vi "Z900_navX_Internal_ProcessingLoop.vi"(11 "navX Device":T1={"Interface"={"Protocol"=enum."SERIAL", "Update Rate (4Hz-100Hz)"=4, "navX Open TypeDef"=variant}, "Notify Packet"=refnum, "Loop VI Refnum"=refnum, "Ready to Close Occurrence Refnum"=refnum} {"Interface"."Update Rate (4Hz-100Hz)" min=4 max=60 step=1}) -> (0 "error out":errorcluster, 2 "Registry":u8[](array[numeric]))   [LabVIEW 2017, in "navX Library v2.lvlib"]
doc: "This navX VI handles the reading/writing for the navX. All of the good stuff is in here.\nTHIS VI SHOULD NOT BE CALLED BY THE USER!"
uses:
  navX Library v2.lvlib
  TypeDefs/Z900_navX_DeviceTypeDef.ctl
  TypeDefs/Z900_navX_ProtocolTypeDef.ctl
  TypeDefs/Z900_navX_NotifyPacketTypeDef.ctl
  TypeDefs/Z900_navX_ActionTypeDef.ctl
  <vilib>/Platform/TimedLoop/XDataNode/timing_clust.ctl
  <vilib>/Platform/TimedLoop/XDataNode/nitl_modes.ctl
  <vilib>/Platform/TimedLoop/XDataNode/wakeup.ctl
  TypeDefs/navX Open TypeDefs/Z900_navX_OpenTypeDef_Serial.ctl
  NI WPI/WPI_SerialPort_USB.ctl
  TypeDefs/Z900_navX_SerialStreamTypeDef.ctl
  TypeDefs/Z900_navX_ZeroVectorTypeDef.ctl
  TypeDefs/Z900_navX_DeviceRegisters.ctl
  TypeDefs/Flags/Z900_navX_Flags_CapabilityTypeDef.ctl
  <vilib>/Rock Robotics/SystemInterfaces/Utilities/FPGA_UtilitiesRead LocalTime.vi
  <vilib>/Platform/TimedLoop/XDataNode/XDataNode.xnode
  <vilib>/Platform/TimedLoop/XDataNode/XDNodeRunTimeDep.lvlib
  NI WPI/NI WPI Serial USB.lvlib
panel:
  out "Connected":bool
  in  "Halt":bool
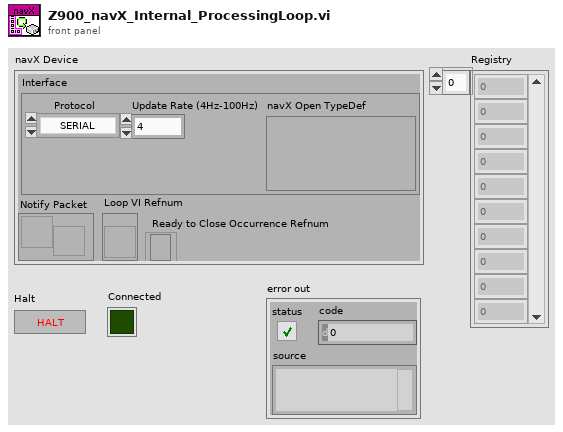
[diagram p1: front panel]
types:
  T1 = typedef "navX Library v2.lvlib/Z900_navX_DeviceTypeDef.ctl" = cluster{"Interface":cluster{"Protocol":T2, "Update Rate (4Hz-100Hz)":u8, "navX Open TypeDef":variant}, "Notify Packet":refnum<notifier>, "Loop VI Refnum":refnum<vi>, "Ready to Close Occurrence Refnum":refnum<k4>}
  T2 = typedef "navX Library v2.lvlib/Z900_navX_ProtocolTypeDef.ctl" = enum16{"SERIAL", "I2C", "SPI"}
  T3 = typedef "navX Library v2.lvlib/Z900_navX_InterfaceTypeDef.ctl" = cluster{"SerialPortRef":T4, "I2CDevRef":T5, "SPIDevRef":T7}
  T4 = typedef "WPI_SerialPortRef.ctl" = cluster{"DevStatus":errorcluster, "Serial Port Name":refnum<visa-resource-name>}
  T5 = typedef "WPI_I2CDevRef.ctl" = cluster{"DevStatus":errorcluster, "Device Address":u8, "Handle":i32, "I2C Bus":T6}
  T6 = typedef "i2c_bus.ctl" = enum16{"I2C On-Board", "I2C MXP", "Invalid"}
  T7 = typedef "WPI_SPIDevRef.ctl" = cluster{"DevStatus":errorcluster, "Handle":i32, "SPI Bus":T8}
  T8 = typedef "spi_bus.ctl" = enum16{"SPI On-Board, CS0", "SPI On-Board, CS1", "SPI On-Board, CS2", "SPI On-Board, CS3", "SPI MXP", "Invalid"}
  T9 = cluster{"Last Valid FPGA Time":dbl, "Error Count":i32, "Initialized":bool}
  T10 = typedef "XDNodeRunTimeDep.lvlib/timing_clust.ctl" = cluster{"Expected End [f-1]":u64, "Actual End [f-1]":u64, "Finished Late? [f-1]":bool, "Expected End [i-1]":u64, "Actual End [i-1]":u64, "Finished Late? [i-1]":bool, "Expected Start [i]":u64, "Actual Start [i]":u64, "Expected Start [f]":u64, "Actual Start [f]":u64, "Source Name":string, "Structure Name":string, "Period":i64, "Deadline":i64, "Offset":i64, "Start":i64, "Priority":i32, "Timeout":i32, "Mode":T11, "Wakeup Reason":T12, "Error":errorcluster, "Source Type":string, "Secondary Source Type":string, "Global End Time":u64, "Global Start Time":u64, "Frame Duration":u64, "Iteration Duration":u64, "Assigned CPU":i32, "I/O Scan Engine Mode":u32}
  T11 = typedef "XDNodeRunTimeDep.lvlib/nitl_modes.ctl" = enum32{"No Change", "Process missed periods, maintain original phase", "Discard missed periods, maintain original phase", "Process missed periods, ignore original phase", "Discard missed periods, ignore original phase"}
  T12 = typedef "XDNodeRunTimeDep.lvlib/wakeup.ctl" = enum32{"Normal", "Aborted", "Asynchronous wakeup", "Timing source error", "Timed loop error", "Timeout"}
  T13 = typedef "navX Library v2.lvlib/Z900_navX_OpenTypeDef_Serial.ctl" = cluster{"Serial Port":T14, "Stream Type":T15}
  T14 = typedef "NI WPI Serial USB.lvlib/WPI_SerialPort_USB.ctl" = enum16{"Onboard RS-232", "MXP TTL", "USB"}
  T15 = typedef "navX Library v2.lvlib/Z900_navX_SerialStreamTypeDef.ctl" = enum16{"YRPH", "Quaterinons", "Gyro/Raw", "AHRS", "AHRSAndPositioning"}
  T16 = typedef "navX Library v2.lvlib/Z900_navX_ZeroVectorTypeDef.ctl" = cluster{"X":bool, "Y":bool, "Z":bool}
  T17 = typedef "navX Library v2.lvlib/Z900_navX_NotifyPacketTypeDef.ctl" = cluster{"navX Action":T18, "Data":variant}
  T18 = typedef "navX Library v2.lvlib/Z900_navX_ActionTypeDef.ctl" = enum16{"None", "Halt", "Update Serial Protocol", "Zero-Yaw", "Zero-Displacement", "Zero-Velocity"}
  T19 = typedef "navX Library v2.lvlib/Z900_navX_DeviceRegisters.ctl" = u8
  T20 = typedef "navX Library v2.lvlib/Z900_navX_Flags_CapabilityTypeDef.ctl" = u16
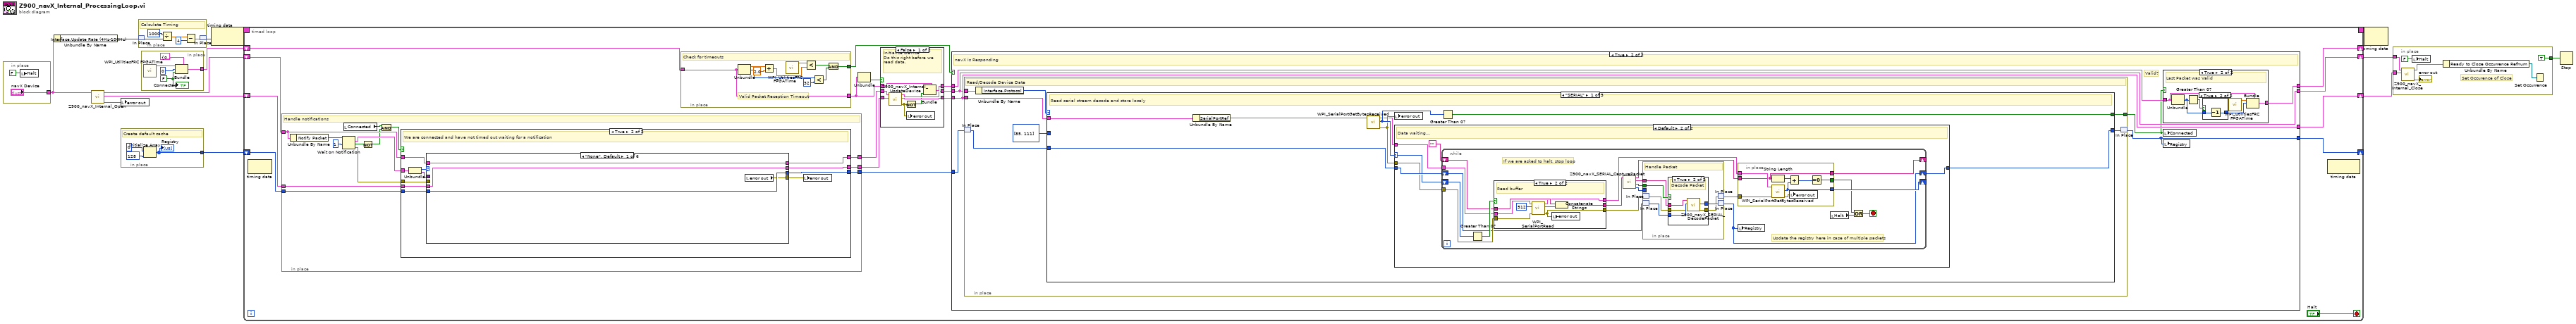
[diagram p0: block diagram]
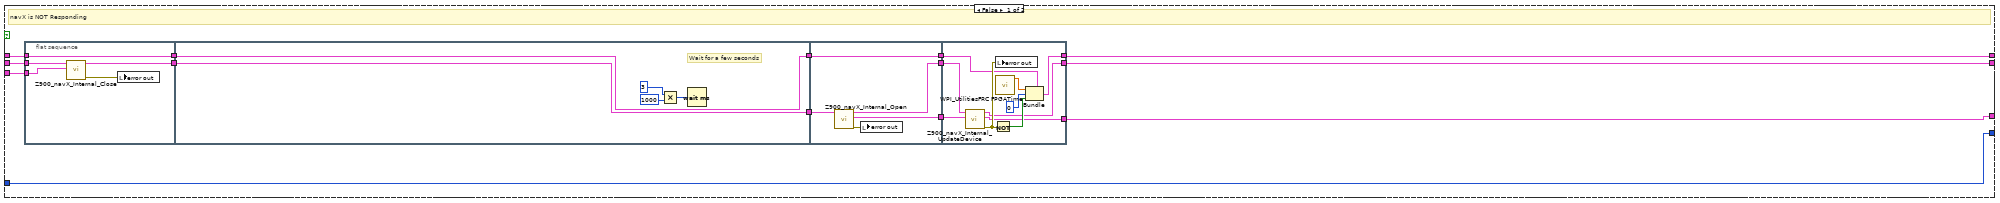
[diagram p3: hidden frame]
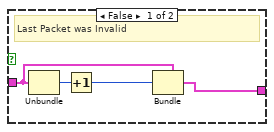
[diagram p4: hidden frame]
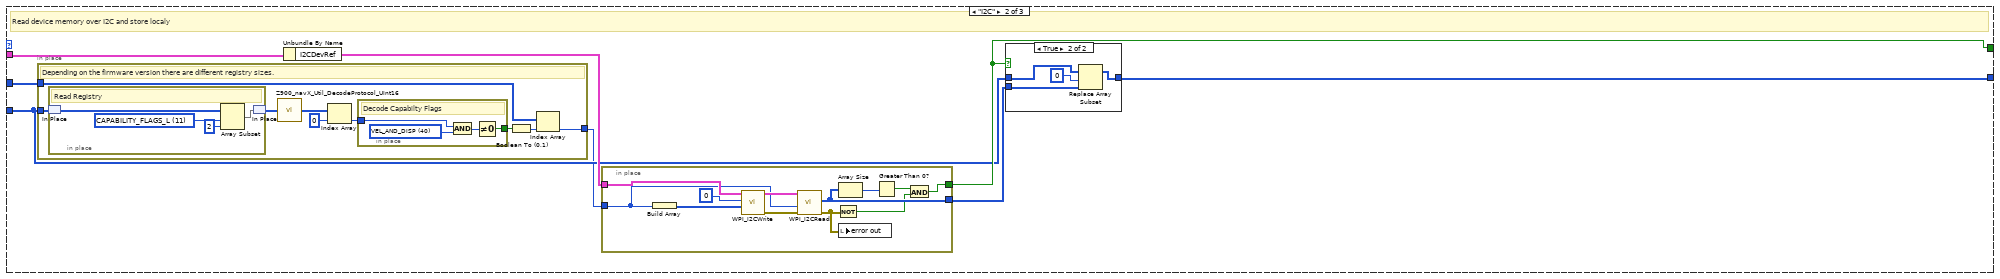
[diagram p9: hidden frame]
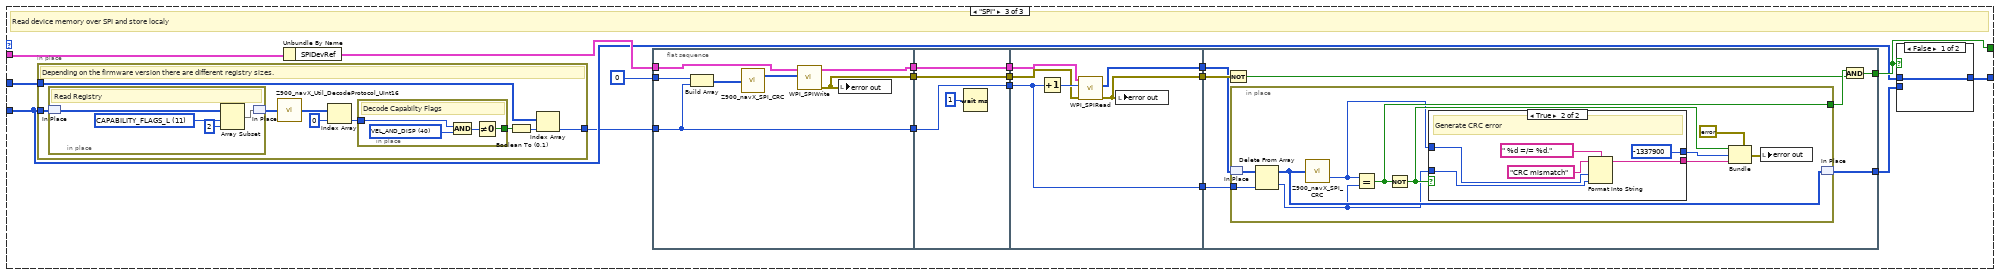
[diagram p11: hidden frame]
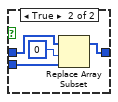
[diagram p12: hidden frame]
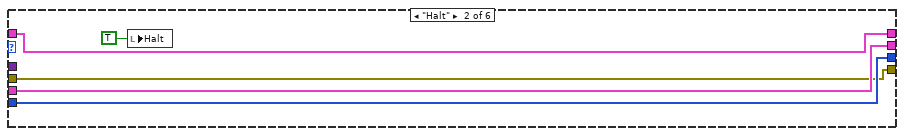
[diagram p15: hidden frame]
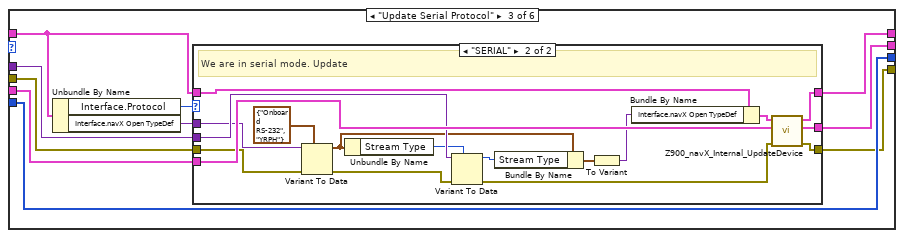
[diagram p16: hidden frame]
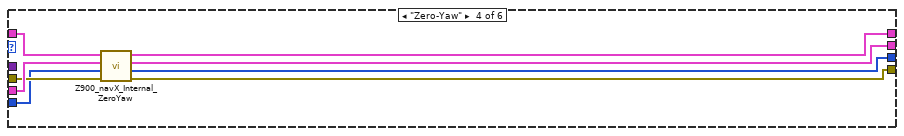
[diagram p18: hidden frame]
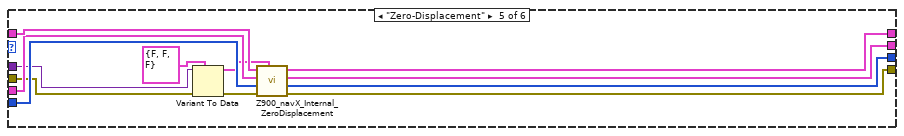
[diagram p19: hidden frame]
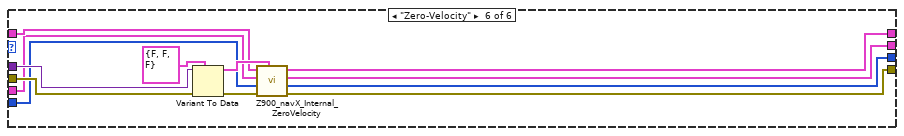
[diagram p20: hidden frame]
diagram:
  n1 = in-place {
    in-place-border: ["navX Device"] -> w6
    n2 = local write "Halt"(FALSE ("Halt")) -> ()
  }
  n3 = Unbundle By Name(w6) -> ("Interface.Update Rate (4Hz-100Hz)"=w10:u8)
  n4 = call "Z900_navX_Internal_Open.vi"("navX Device"=w6) -> ("error out"=w2:errorcluster, "Interface TypeDefs"=w5:T3, "navX Device"=w3:T1)  [unwired: 8 in]
  n5 = local write "error out"(w2) -> ()
  n6 = in-place {
    in-place-border: [w16] -> w9
    # "Create default cache"
    n7 = Initialize Array(u8 0 ("Received Data"), 128 ("hex")) -> (w16:u8[])
    "Registry" <- w16
  }
  n8 = in-place {
    # "Calculate Timing"
    n9 = in-place-match #1(w10) -> (w22:u8)
    n10 = Divide(x=1000, y=w22) -> (x/y=w20:dbl)
    n11 = Subtract(x=w20, y=4) -> (x-y=w19:dbl)
    n12 = in-place-match #1(w19) -> (w11:u8)
  }
  n13 = in-place {
    in-place-border: [w26] -> w4
    w24 = FALSE ("Initialized")
    n14 = call <vilib>:"WPI_UtilitiesFRC FPGATime.vi"() -> ("FPGA Time"=w27:dbl)  [unwired: 10 in, 1 out]
    n15 = Bundle(cluster=T9 {"Last Valid FPGA Time"=0.0, "Error Count"=0, "Initialized"=FALSE}, "Last Valid FPGA Time"=w27, "Error Count"=0, "Initialized"=w24) -> (w26:T9)
    "Connected" <- w24
  }
  n16 = node-c288(w11) -> (w13:T10)
  n17 = timed-loop {
    timing: w13 -> [_]
    timing-out: [_] -> w12
    shift-right: [w46] -> _
    shift-left: w9 -> [w42]
    shift-right: [w43] -> w8
    shift-left: w3 -> [w32]
    shift-right: [w44] -> w7
    shift-left: w5 -> [w31]
    shift-right: [w45] -> _
    shift-left: w4 -> [w29]
    stop <- "Halt" stop-if-true
    n18 = node-c288() -> ()  [unwired: 1 in, 1 out]
    n19 = in-place {
      in-place-border: w32 -> [w334]
      in-place-border: w31 -> [w333]
      in-place-border: [w332] -> w35
      in-place-border: [w331] -> w36
      in-place-border: w42 -> [w329]
      in-place-border: [w328] -> w41
      # "Handle notifications"
      n20 = Unbundle By Name(w334) -> ("Notify Packet"=w336:refnum<notifier>)
      n21 = Wait on Notification(notifier=w336, timeout in ms (-1)=1) -> (notification=w337:T17, timed out?=w327:bool, error out=w330:errorcluster)  [unwired: 2 in, 1 out]
      n22 = local read "Connected"() -> (w325:bool)
      n23 = Not(x=w327) -> (.not. x?=w326:bool)
      n24 = And(x=w325, y=w326) -> (x .and. y?=w324:bool)
      n25 = case shown="True" w324 {
        tunnel: w337 -> [_ w351]
        tunnel: w334 -> [w340 w349]
        tunnel: w333 -> [w339 w348]
        tunnel: [w339 w347] -> w332
        tunnel: [w340 w346] -> w331
        tunnel: w330 -> [_ w344]
        tunnel: w329 -> [w338 w343]
        tunnel: [w338 w342] -> w328
        frame False {
          # "We are either not connected or have timed out waiting for a notification"
        }
        frame True {
          # "We are connected and have not timed out waiting for a notification"
          n26 = Unbundle(w351) -> ("navX Action"=w350:T18, "Data"=w345:variant)
          n27 = case shown="\"None\", Default" w350 {
            tunnel: w349 -> [w355 w360 w364 w398 w410 w417]
            tunnel: w348 -> [w354 w359 w370 w396 w408 w416]
            tunnel: [w354 w359 w369 w395 w406 w413] -> w347
            tunnel: [w355 w360 w368 w397 w407 w414] -> w346
            tunnel: w345 -> [_ _ w367 _ w403 w420]
            tunnel: w344 -> [_ w357 w365 w394 w400 w421]
            tunnel: w343 -> [w353 w358 w363 w393 w409 w415]
            tunnel: [w353 w358 w363 w392 w405 w412] -> w342
            tunnel: [w352 w357 w362 w391 w404 w411] -> w341
            frame "None", Default {
              n28 = local read "error out"() -> (w352:errorcluster)
            }
            frame "Halt" {
              n29 = local write "Halt"(TRUE) -> ()
            }
            frame "Update Serial Protocol" {
              n30 = Unbundle By Name(w364) -> ("Interface.Protocol"=w361:T2, "Interface.navX Open TypeDef"=w366:variant)
              n31 = case shown="\"SERIAL\"" w361 {
                tunnel: w370 -> [w372 w390]
                tunnel: [w372 w389] -> w369
                tunnel: [w373 w388] -> w368
                tunnel: w367 -> [_ w387]
                tunnel: w366 -> [_ w384]
                tunnel: w365 -> [w371 w381]
                tunnel: w364 -> [w373 w380]
                tunnel: [w371 w374] -> w362
                frame Default {
                  # "We don't care if we are not in serial mode."
                }
                frame "SERIAL" {
                  # "We are in serial mode. Update"
                  n32 = Variant To Data(error in=w381, type=T13 {"Serial Port"=enum."Onboard RS-232", "Stream Type"=enum."YRPH"} ("navX Serial Open"), Variant=w384) -> (data=w377:T13, error out=w382:errorcluster)
                  n33 = Unbundle By Name(w377) -> ("Stream Type"=w376:T15)
                  n34 = Variant To Data(error in=w382, type=w376, Variant=w387) -> (data=w375:T15, error out=w386:errorcluster)
                  n35 = Bundle By Name(cluster=w377, "Stream Type"=w375) -> (w385:T13)
                  n36 = To Variant(anything=w385) -> (Variant=w379:variant)
                  n37 = Bundle By Name(cluster=w380, "Interface.navX Open TypeDef"=w379) -> (w378:T1)
                  n38 = call "Z900_navX_Internal_UpdateDevice.vi"("error in (no error)"=w386, "Interface TypeDefs"=w390, "navX Device"=w378) -> ("error out"=w374:errorcluster, "Interface TypeDefs"=w389:T3, "navX Device"=w388:T1)  [unwired: 6 in]
                }
              }
            }
            frame "Zero-Yaw" {
              n39 = call "Z900_navX_Internal_ZeroYaw.vi"("error in (no error)"=w394, "Registry"=w393, "Interface TypeDefs"=w396, "navX Device"=w398) -> ("error out"=w391:errorcluster, "Registry"=w392:u8[], "Interface TypeDefs"=w395:T3, "navX Device"=w397:T1)  [unwired: 4 in]
            }
            frame "Zero-Displacement" {
              n40 = Variant To Data(error in=w400, type=T16 {"X"=FALSE, "Y"=FALSE, "Z"=FALSE} ("Zero Vector"), Variant=w403) -> (data=w401:T16, error out=w399:errorcluster)
              n41 = call "Z900_navX_Internal_ZeroDisplacement.vi"("Zero Vector"=w401, "error in (no error)"=w399, "Registry"=w409, "Interface TypeDefs"=w408, "navX Device"=w410) -> ("error out"=w404:errorcluster, "Registry"=w405:u8[], "Interface TypeDefs"=w406:T3, "navX Device"=w407:T1)  [unwired: 3 in]
            }
            frame "Zero-Velocity" {
              n42 = Variant To Data(error in=w421, type=T16 {"X"=FALSE, "Y"=FALSE, "Z"=FALSE} ("Zero Vector"), Variant=w420) -> (data=w419:T16, error out=w418:errorcluster)
              n43 = call "Z900_navX_Internal_ZeroVelocity.vi"("Zero Vector"=w419, "error in (no error)"=w418, "Registry"=w415, "Interface TypeDefs"=w416, "navX Device"=w417) -> ("error out"=w411:errorcluster, "Registry"=w412:u8[], "Interface TypeDefs"=w413:T3, "navX Device"=w414:T1)  [unwired: 3 in]
            }
          }
          n44 = local write "error out"(w341) -> ()
        }
      }
    }
    n45 = in-place {
      in-place-border: w29 -> [w58]
      in-place-border: [w59] -> w40
      in-place-border: [w58] -> w30
      # "Valid Packet Reception Timeout"
      # "Check for timeouts"
      n46 = Unbundle(w58) -> ("Last Valid FPGA Time"=w67:dbl, "Error Count"=w63:i32)  [unwired: 1 out]
      n47 = Add(x=w67, y=2.0) -> (x+y=w65:dbl)
      n48 = call <vilib>:"WPI_UtilitiesFRC FPGATime.vi"() -> ("FPGA Time"=w64:dbl)  [unwired: 10 in, 1 out]
      n49 = Less?(x=w64, y=w65) -> (x < y?=w61:bool)
      n50 = Less?(x=w63, y=32) -> (x < y?=w60:bool)
      n51 = And(x=w61, y=w60) -> (x .and. y?=w59:bool)
    }
    n52 = Unbundle(w30) -> ("Initialized"=w38:bool)  [unwired: 2 out]
    n53 = case shown="False" w38 {
      tunnel: w30 -> [w54 w57]
      tunnel: [w53 w57] -> w37
      tunnel: w36 -> [w52 w56]
      tunnel: w35 -> [w51 w55]
      tunnel: [w50 w56] -> w33
      tunnel: [w49 w55] -> w34
      frame False {
        # "Initialize Device\nDo this right before we\nread data."
        n54 = call "Z900_navX_Internal_UpdateDevice.vi"("Interface TypeDefs"=w51, "navX Device"=w52) -> ("error out"=w48:errorcluster, "Interface TypeDefs"=w49:T3, "navX Device"=w50:T1)  [unwired: 7 in]
        n55 = Not(x=w48) -> (.not. x?=w47:bool)
        n56 = local write "error out"(w48) -> ()
        n57 = Bundle(cluster=w54, "Initialized"=w47) -> (w53:T9)  [unwired: 2 in]
      }
      frame True {
      }
    }
    n58 = case shown="True" w40 {
      tunnel: w41 -> [w79 w113]
      tunnel: w34 -> [w80 w112]
      tunnel: [w79 w109] -> w46
      tunnel: w37 -> [w68 w111]
      tunnel: [w72 w110] -> w45
      tunnel: w33 -> [w81 w108]
      tunnel: [w73 w108] -> w43
      tunnel: [w76 w112] -> w44
      frame False {
        # "navX is NOT Responding"
        n59 = flat-sequence {
          tunnel: w81 -> [w84]
          tunnel: w80 -> [w86]
          tunnel: [w85] -> w78
          tunnel: [w82] -> w69
          tunnel: w68 -> [w82]
          tunnel: w78 -> [w91]
          tunnel: [w91] -> w77
          tunnel: [w87] -> w70
          tunnel: w69 -> [w87]
          tunnel: w77 -> [w95]
          tunnel: [w96] -> w75
          tunnel: [w94] -> w74
          tunnel: [w92] -> w71
          tunnel: w70 -> [w92]
          tunnel: [w104] -> w72
          tunnel: [w100] -> w76
          tunnel: [w101] -> w73
          tunnel: w71 -> [w99]
          tunnel: w74 -> [w102]
          tunnel: w75 -> [w103]
          frame #0 {
            n60 = call "Z900_navX_Internal_Close.vi"("Interface TypeDefs"=w86, "navX Device"=w84) -> ("error out"=w83:errorcluster, "navX Device"=w85:T1)  [unwired: 8 in]
            n61 = local write "error out"(w83) -> ()
          }
          frame #1 {
            # "Wait for a few seconds"
            n62 = Multiply(x=u32 3 ("milliseconds to wait"), y=u32 1000) -> (x*y=w89:u32)
            n63 = Wait (ms)(milliseconds to wait=w89) -> ()  [unwired: 1 out]
          }
          frame #2 {
            n64 = call "Z900_navX_Internal_Open.vi"("navX Device"=w95) -> ("error out"=w93:errorcluster, "Interface TypeDefs"=w94:T3, "navX Device"=w96:T1)  [unwired: 8 in]
            n65 = local write "error out"(w93) -> ()
          }
          frame #3 {
            n66 = call "Z900_navX_Internal_UpdateDevice.vi"("Interface TypeDefs"=w102, "navX Device"=w103) -> ("error out"=w105:errorcluster, "Interface TypeDefs"=w100:T3, "navX Device"=w101:T1)  [unwired: 7 in]
            n67 = Not(x=w105) -> (.not. x?=w106:bool)
            n68 = local write "error out"(w105) -> ()
            n69 = call <vilib>:"WPI_UtilitiesFRC FPGATime.vi"() -> ("FPGA Time"=w98:dbl)  [unwired: 10 in, 1 out]
            n70 = Bundle(cluster=w99, "Last Valid FPGA Time"=w98, "Error Count"=0, "Initialized"=w106) -> (w104:T9)
          }
        }
      }
      frame True {
        # "Valid?"
        # "navX is Responding"
        n71 = in-place {
          in-place-border: w108 -> [w128]
          in-place-border: w112 -> [w132]
          in-place-border: [w130] -> w107
          # "Read/Decode Device Date"
          n72 = in-place-match #2(w113) -> (w131:u8[])
          n73 = Unbundle By Name(w128) -> ("Interface.Protocol"=w133:T2)
          n74 = case shown="\"SERIAL\"" w133 {
            tunnel: [w139 w206 w253] -> w129
            tunnel: w131 -> [w140 w203 w245]
            tunnel: w132 -> [w141 w208 w260]
            tunnel: [w137 w205 w250] -> w130
            tunnel: i32[] [85, 111] -> [_ w202 w244]
            frame "SERIAL" {
              # "Read serial stream decode and store localy"
              n75 = Unbundle By Name(w141) -> ("SerialPortRef"=w138:T4)
              n76 = call <vilib>:"WPI_SerialPortGetBytesReceived.vi"("SerialPortRef"=w138) -> ("error out"=w135:errorcluster, "Bytes at Port"=w136:u32, "SerialPortRef"=w134:T4)  [unwired: 8 in]
              n77 = local write "error out"(w135) -> ()
              n78 = case shown="Default" w136 {
                selector: w136 -> [_ w143]
                tunnel: [w142 w148] -> w139
                tunnel: w140 -> [w142 w147]
                tunnel: w134 -> [_ w145]
                tunnel: w135 -> [_ w144]
                frame 0 {
                }
                frame Default {
                  # "Data waiting..."
                  n79 = while {
                    shift-right: [w150] -> w148
                    shift-left: w147 -> [w157]
                    shift-right: [w161] -> _
                    shift-left: w143 -> [w168]
                    shift-right: [w160] -> _
                    shift-left: "" -> [w166]
                    tunnel: w145 -> [w165]
                    tunnel: w144 -> [w164]
                    stop <- w153 stop-if-true
                    # "Update the registry here in case of multiple packets"
                    # "If we are asked to halt, stop loop"
                    n80 = Greater Than 0?(x=w168) -> (x > 0?=w167:bool)
                    n81 = case shown="True" w167 {
                      tunnel: w166 -> [w192 w200]
                      tunnel: w165 -> [w191 w199]
                      tunnel: w164 -> [w190 w196]
                      tunnel: [w192 w195] -> w163
                      tunnel: [w191 w194] -> w149
                      tunnel: [w190 w193] -> w156
                      frame False {
                        # "Pass existing buffer"
                      }
                      frame True {
                        # "Read buffer"
                        n82 = call <vilib>:"WPI_SerialPortRead.vi"("error in (no error)"=w196, "Num Bytes to Read"=u32 512, "SerialPortRef"=w199) -> ("error out"=w193:errorcluster, "Buffer"=w198:string, "SerialPortRef"=w194:T4)  [unwired: 6 in]
                        n83 = local write "error out"(w193) -> ()
                        n84 = Concatenate Strings(w200, w198) -> (w195:string)
                      }
                    }
                    n85 = call "Z900_navX_SERIAL_CapturePacket.vi"("Buffer"=w163) -> ("Packet Size"=w158:i32, "Packet Located"=w151:bool, "Packet"=w159:string, "Buffer"=w162:string)  [unwired: 7 in]
                    n86 = in-place {
                      in-place-border: w159 -> [w173]
                      in-place-border: w151 -> [w174]
                      in-place-border: w158 -> [_]
                      # "Handle Packet"
                      n87 = in-place-match #3(w156) -> (w170:errorcluster)
                      n88 = in-place-match #4(w157) -> (w171:u8[])
                      n89 = case shown="True" w174 {
                        tunnel: w173 -> [_ w181]
                        tunnel: [w176 w179] -> w172
                        tunnel: w171 -> [w176 w180]
                        tunnel: w170 -> [w175 w178]
                        tunnel: [w175 w177] -> w169
                        frame False {
                          # "No Packet"
                        }
                        frame True {
                          # "Decode Packet"
                          n90 = call "Z900_navX_SERIAL_DecodePacket.vi"("error in (no error)"=w178, "Data"=w180, "Packet"=w181) -> ("error out"=w177:errorcluster, "Data"=w179:u8[])  [unwired: 6 in, 1 out]
                        }
                      }
                      n91 = in-place-match #3(w169) -> (w155:errorcluster)
                      n92 = in-place-match #4(w172) -> (w150:u8[])
                    }
                    n93 = in-place {
                      in-place-border: w149 -> [w189]
                      in-place-border: w155 -> [w188]
                      in-place-border: w162 -> [w183]
                      in-place-border: [w185] -> w154
                      in-place-border: [w184] -> w161
                      in-place-border: [w183] -> w160
                      n94 = String Length(string=w183) -> (length=w186:i32)
                      n95 = call <vilib>:"WPI_SerialPortGetBytesReceived.vi"("error in (no error)"=w188, "SerialPortRef"=w189) -> ("error out"=w182:errorcluster, "Bytes at Port"=w184:u32)  [unwired: 7 in, 1 out]
                      n96 = Add(x=w186, y=w184) -> (x+y=w187:u32)
                      n97 = local write "error out"(w182) -> ()
                      n98 = Equal To 0?(x=w187) -> (x = 0?=w185:bool)
                    }
                    n99 = local write "Registry"(w150) -> ()
                    n100 = local read "Halt"() -> (w152:bool)
                    n101 = Or(x=w154, y=w152) -> (x .or. y?=w153:bool)
                  }
                }
              }
              n102 = Greater Than 0?(x=w136) -> (x > 0?=w137:bool)
            }
            frame "I2C" {
              # "Read device memory over I2C and store localy"
              n103 = in-place {
                in-place-border: w203 -> [w217]
                in-place-border: w202 -> [w210]
                in-place-border: [w209] -> w201
                # "Depending on the firmware version there are different registry sizes."
                n104 = in-place {
                  w225 = T19 11 items=["WHOAMI"=0, "HW_REV"=1, "FW_VER_MAJOR"=2, "FW_VER_MINOR"=3, "UPDATE_RATE_HZ"=4, "ACCEL_FSR_G"=5, "GYRO_FSR_DPS"=6, "OP_STATUS"=8, "CAL_STATUS"=9, "SELFTEST_STATUS"=10, "CAPABILITY_FLAGS_L"=11, "CAPABILITY_FLAGS_H"=12, "SENSOR_STATUS"=16, "TIMESTAMP"=18, "YAW"=22, "ROLL"=24, "PITCH"=26, "HEADING"=28, "FUSED_HEADING"=30, "ALTITUDE_I"=32, "ALTITUDE_D"=34, "LINERA_ACC_X"=36, "LINERA_ACC_Y"=38, "LINERA_ACC_Z"=40, "QUAT_W"=42, "QUAT_X"=44, "QUAT_Y"=46, "QUAT_Z"=48, "MPU_TEMP_C"=50, "GYRO_X"=52, "GYRO_Y"=54, "GYRO_Z"=56, "ACC_X"=58, "ACC_Y"=60, "ACC_Z"=62, "MAG_X"=64, "MAG_Y"=66, "MAG_Z"=68, "PRESSURE_I"=70, "PRESSURE_D"=72, "PRESSURE_TEMP"=74, "YAW_OFFSET"=76, "QUAT_OFFSET_W"=78, "QUAT_OFFSET_X"=80, "QUAT_OFFSET_Y"=82, "QUAT_OFFSET_Z"=84, "INTEGRATION_CONTROL"=86, "VELOCITY_X"=88, "VELOCITY_Y"=92, "VELOCITY_Z"=96, "DISPLACMENT_X"=100, "DISPLACMENT_Y"=104, "DISPLACEMENT_Z"=108] ("Device Register")
                  # "Read Registry"
                  n105 = in-place-match #5(w217) -> (w223:u8[])
                  n106 = Array Subset(array=w223, index=w225, length=2) -> (w224:u8[])
                  n107 = in-place-match #5(w224) -> (w214:u8[])
                }
                n108 = call "Z900_navX_Util_DecodeProtocol_UInt16.vi"("Little Endian"=w214) -> ("UInt16"=w215:u16[])
                n109 = Index Array(array=w215, index=0) -> (element=w213:u16)
                n110 = in-place {
                  in-place-border: w213 -> [w219]
                  in-place-border: [w218] -> w212
                  w221 = T20 40 items=["OMNIMOUNT"=4, "OMNIMOUNT_CONFIG_MASK"=38, "VEL_AND_DISP"=40, "YAW_RESET"=80] ("Capability Flag")
                  # "Decode Capabilty Flags"
                  n111 = And(x=w219, y=w221) -> (x .and. y?=w220:T20)
                  n112 = Not Equal To 0?(x=w220) -> (x != 0?=w218:bool)
                }
                n113 = Boolean To (0,1)(Boolean=w212) -> (0, 1=w211:i16)
                n114 = Index Array(array=w210, index=w211) -> (element=w209:i32)
              }
              n115 = Unbundle By Name(w208) -> ("I2CDevRef"=w204:T5)
              n116 = in-place {
                in-place-border: [w231] -> w207
                in-place-border: [w230] -> w205
                in-place-border: w204 -> [w228]
                in-place-border: w201 -> [w226]
                n117 = Build Array(w226) -> (w237:i32[])
                n118 = call <vilib>:"WPI_I2CWrite.vi"("I2CDataToSend"=w237, "I2CRegister"=u8 0 ("hex"), "I2CDevRef"=w228) -> ("error out"=w236:errorcluster, "I2CDevRef"=w235:T5)  [unwired: 7 in]
                n119 = call <vilib>:"WPI_I2CRead.vi"("error in (no error)"=w236, "I2CBytesToRead"=w226, "I2CDevRef"=w235) -> ("error out"=w227:errorcluster, "Data Out"=w231:u8[])  [unwired: 6 in, 1 out]
                n120 = Not(x=w227) -> (.not. x?=w229:bool)
                n121 = Array Size(array=w231) -> (size(s)=w233:i32)
                n122 = local write "error out"(w227) -> ()
                n123 = Greater Than 0?(x=w233) -> (x > 0?=w232:bool)
                n124 = And(x=w232, y=w229) -> (x .and. y?=w230:bool)
              }
              n125 = case shown="True" w205 {
                tunnel: w203 -> [w238 w242]
                tunnel: [w238 w241] -> w206
                tunnel: w207 -> [_ w240]
                frame False {
                }
                frame True {
                  n126 = Replace Array Subset(array=w242, new element=w240, index=u8 0 ("hex")) -> (w241:u8[])
                }
              }
            }
            frame "SPI" {
              # "Read device memory over SPI and store localy"
              n127 = in-place {
                in-place-border: w245 -> [w269]
                in-place-border: w244 -> [w262]
                in-place-border: [w261] -> w243
                # "Depending on the firmware version there are different registry sizes."
                n128 = in-place {
                  w277 = T19 11 items=["WHOAMI"=0, "HW_REV"=1, "FW_VER_MAJOR"=2, "FW_VER_MINOR"=3, "UPDATE_RATE_HZ"=4, "ACCEL_FSR_G"=5, "GYRO_FSR_DPS"=6, "OP_STATUS"=8, "CAL_STATUS"=9, "SELFTEST_STATUS"=10, "CAPABILITY_FLAGS_L"=11, "CAPABILITY_FLAGS_H"=12, "SENSOR_STATUS"=16, "TIMESTAMP"=18, "YAW"=22, "ROLL"=24, "PITCH"=26, "HEADING"=28, "FUSED_HEADING"=30, "ALTITUDE_I"=32, "ALTITUDE_D"=34, "LINERA_ACC_X"=36, "LINERA_ACC_Y"=38, "LINERA_ACC_Z"=40, "QUAT_W"=42, "QUAT_X"=44, "QUAT_Y"=46, "QUAT_Z"=48, "MPU_TEMP_C"=50, "GYRO_X"=52, "GYRO_Y"=54, "GYRO_Z"=56, "ACC_X"=58, "ACC_Y"=60, "ACC_Z"=62, "MAG_X"=64, "MAG_Y"=66, "MAG_Z"=68, "PRESSURE_I"=70, "PRESSURE_D"=72, "PRESSURE_TEMP"=74, "YAW_OFFSET"=76, "QUAT_OFFSET_W"=78, "QUAT_OFFSET_X"=80, "QUAT_OFFSET_Y"=82, "QUAT_OFFSET_Z"=84, "INTEGRATION_CONTROL"=86, "VELOCITY_X"=88, "VELOCITY_Y"=92, "VELOCITY_Z"=96, "DISPLACMENT_X"=100, "DISPLACMENT_Y"=104, "DISPLACEMENT_Z"=108] ("Device Register")
                  # "Read Registry"
                  n129 = in-place-match #6(w269) -> (w275:u8[])
                  n130 = Array Subset(array=w275, index=w277, length=2) -> (w276:u8[])
                  n131 = in-place-match #6(w276) -> (w266:u8[])
                }
                n132 = call "Z900_navX_Util_DecodeProtocol_UInt16.vi"("Little Endian"=w266) -> ("UInt16"=w267:u16[])
                n133 = Index Array(array=w267, index=0) -> (element=w265:u16)
                n134 = in-place {
                  in-place-border: w265 -> [w271]
                  in-place-border: [w270] -> w264
                  w273 = T20 40 items=["OMNIMOUNT"=4, "OMNIMOUNT_CONFIG_MASK"=38, "VEL_AND_DISP"=40, "YAW_RESET"=80] ("Capability Flag")
                  # "Decode Capabilty Flags"
                  n135 = And(x=w271, y=w273) -> (x .and. y?=w272:T20)
                  n136 = Not Equal To 0?(x=w272) -> (x != 0?=w270:bool)
                }
                n137 = Boolean To (0,1)(Boolean=w264) -> (0, 1=w263:i16)
                n138 = Index Array(array=w262, index=w263) -> (element=w261:i32)
              }
              n139 = Unbundle By Name(w260) -> ("SPIDevRef"=w246:T7)
              n140 = flat-sequence {
                tunnel: u8 0 ("hex") -> [w289]
                tunnel: w243 -> [w284]
                tunnel: w246 -> [w286]
                tunnel: [w285] -> w259
                tunnel: [w284] -> w256
                tunnel: [w283] -> w249
                tunnel: w259 -> [w292]
                tunnel: [w292] -> w258
                tunnel: [w291] -> w257
                tunnel: w256 -> [w291]
                tunnel: w249 -> [w290]
                tunnel: [w290] -> w248
                tunnel: w258 -> [w299]
                tunnel: w257 -> [w296]
                tunnel: [w297] -> w255
                tunnel: [w296] -> w254
                tunnel: w248 -> [w295]
                tunnel: [w294] -> w247
                tunnel: w255 -> [w302]
                tunnel: w254 -> [w306]
                tunnel: [w303] -> w250
                tunnel: [w301] -> w252
                tunnel: w247 -> [w305]
                frame #0 {
                  n141 = Build Array(w289, w284) -> (w288:i32[])
                  n142 = call "Z900_navX_SPI_CRC.vi"("Message"=w288) -> ("Message with CRC"=w287:u8[])  [unwired: 1 out]
                  n143 = call <vilib>:"WPI_SPIWrite.vi"("Data To Send"=w287, "SPIDevRef"=w286) -> ("error out"=w283:errorcluster, "SPIDevRef"=w285:T7)  [unwired: 7 in, 1 out]
                  n144 = local write "error out"(w283) -> ()
                }
                frame #1 {
                  n145 = Wait (ms)(milliseconds to wait=u32 1) -> ()  [unwired: 1 out]
                }
                frame #2 {
                  n146 = Increment(x=w296) -> (x+1=w298:i32)
                  n147 = call <vilib>:"WPI_SPIRead.vi"("error in (no error)"=w295, "Num to Read"=w298, "SPIDevRef"=w299) -> ("error out"=w294:errorcluster, "Received Data"=w297:u8[])  [unwired: 6 in, 1 out]
                  n148 = local write "error out"(w294) -> ()
                }
                frame #3 {
                  n149 = Not(x=w305) -> (.not. x?=w300:bool)
                  n150 = in-place {
                    in-place-border: w306 -> [w317]
                    in-place-border: [w314] -> w304
                    n151 = in-place-match #7(w302) -> (w316:u8[])
                    n152 = Delete From Array(array=w316, index=w317) -> (deleted portion=w311:u8, array with subset deleted=w315:u8[])  [unwired: 1 in]
                    n153 = call "Z900_navX_SPI_CRC.vi"("Message"=w315) -> ("CRC"=w312:u8)  [unwired: 1 out]
                    n154 = Equal?(x=w312, y=w311) -> (x = y?=w314:bool)
                    n155 = Not(x=w314) -> (.not. x?=w313:bool)
                    n156 = case shown="True" w313 {
                      tunnel: w312 -> [_ w321]
                      tunnel: w311 -> [_ w320]
                      tunnel: [_ w319] -> w310
                      tunnel: [_ -1337900 ("code")] -> w307
                      frame False {
                      }
                      frame True {
                        # "Generate CRC error"
                        n157 = Format Into String(format string=" %d =/= %d.", initial string="CRC mismatch", w321, w320) -> (resulting string=w319:string)  [unwired: 1 in, 1 out]
                      }
                    }
                    n158 = Bundle(cluster=errorcluster {"status"=FALSE, "code"=0, "source"=""} ("error constant"), "status"=w313, "code"=w307, "source"=w310) -> (w308:errorcluster)
                    n159 = local write "error out"(w308) -> ()
                    n160 = in-place-match #7(w315) -> (w301:u8[])
                  }
                  n161 = And(x=w304, y=w300) -> (x .and. y?=w303:bool)
                }
              }
              n162 = case shown="False" w250 {
                tunnel: w245 -> [w278 w282]
                tunnel: [w278 w281] -> w253
                tunnel: w252 -> [_ w280]
                frame False {
                }
                frame True {
                  n163 = Replace Array Subset(array=w282, new element=w280, index=u8 0 ("hex")) -> (w281:u8[])
                }
              }
            }
          }
          n164 = in-place-match #2(w129) -> (w109:u8[])
        }
        n165 = case shown="True" w107 {
          tunnel: [w114 w122] -> w110
          tunnel: w111 -> [w115 w121]
          frame False {
            # "Last Packet was Invalid"
            n166 = Unbundle(w115) -> ("Error Count"=w116:i32)  [unwired: 2 out]
            n167 = Increment(x=w116) -> (x+1=w117:i32)
            n168 = Bundle(cluster=w115, "Error Count"=w117) -> (w114:T9)  [unwired: 2 in]
          }
          frame True {
            # "Last Packet was Valid"
            n169 = Unbundle(w121) -> ("Error Count"=w119:i32)  [unwired: 2 out]
            n170 = Greater Than 0?(x=w119) -> (x > 0?=w120:bool)
            n171 = case shown="True" w120 {
              tunnel: [w124 w125] -> w118
              tunnel: w119 -> [w124 w126]
              frame False {
              }
              frame True {
                n172 = Decrement(x=w126) -> (x-1=w125:i32)
              }
            }
            n173 = call <vilib>:"WPI_UtilitiesFRC FPGATime.vi"() -> ("FPGA Time"=w123:dbl)  [unwired: 10 in, 1 out]
            n174 = Bundle(cluster=w121, "Last Valid FPGA Time"=w123, "Error Count"=w118) -> (w122:T9)  [unwired: 1 in]
          }
        }
        n175 = local write "Connected"(w107) -> ()
        n176 = local write "Registry"(w109) -> ()
      }
    }
    n177 = node-c288() -> ()  [unwired: 1 in, 1 out]
  }
  n178 = node-c288(w12) -> ()  [unwired: 1 out]
  n179 = in-place {
    in-place-border: w8 -> [w431]
    in-place-border: w7 -> [w430]
    in-place-border: [TRUE] -> w1
    # "Set Occurence of Close"
    n180 = call "Z900_navX_Internal_Close.vi"("Interface TypeDefs"=w430, "navX Device"=w431) -> ("error out"=→"error out":errorcluster, "navX Device"=w425:T1)  [unwired: 8 in]
    n181 = local write "Halt"(FALSE ("Halt")) -> ()
    n182 = Unbundle By Name(w425) -> ("Ready to Close Occurrence Refnum"=w427:refnum<k4>)
    n183 = Set Occurrence(w427) -> ()
  }
  n184 = Stop(stop? (T)=w1) -> ()
